vi "Format.vi"(8 "error in (no error)":errorcluster, 10 "LogRecord":refnum<class "LogRecord.lvclass">, 11 "DefaultLogFormat in":refnum<class "DefaultLogFormat.lvclass">) -> (0 "error out":errorcluster, 2 "Log Line":string, 3 "DefaultLogFormat out":refnum<class "DefaultLogFormat.lvclass">)   [LabVIEW 2024, in "DefaultLogFormat.lvclass"]
uses:
  DefaultLogFormat.lvclass
  Record/LogRecord.lvclass
  Record/LogRecord.lvclass/LogRecord.ctl
  DefaultLogFormat.lvclass/DefaultLogFormat.ctl
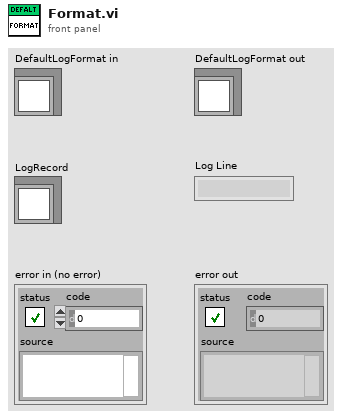
[diagram p1: front panel]
types:
  T1 = typedef "LoggerShared.lvlib/Level.ctl" = enum16{"DEBUG", "INFO", "WARNING", "ERROR", "CRITICAL"}
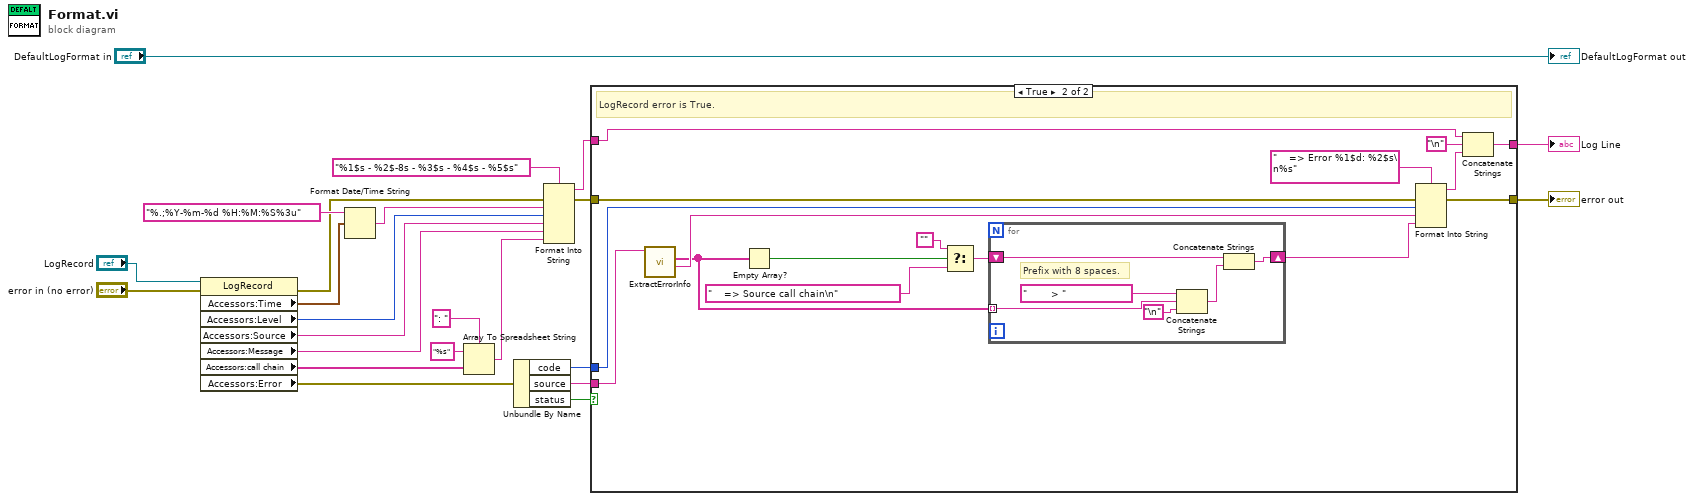
[diagram p0: block diagram]
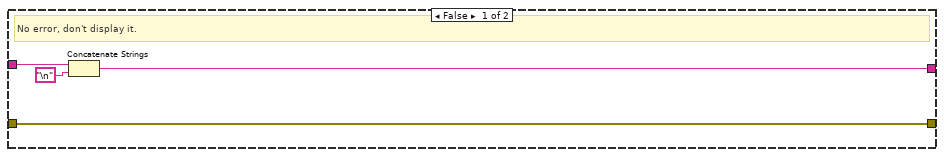
[diagram p2: hidden frame]
diagram:
  n1 = property class="LogRecord"(reference="LogRecord", error in="error in (no error)") -> (error out=w3:errorcluster, "Accessors:Time"=w20:timestamp, "Accessors:Level"=w17:T1, "Accessors:Source"=w16:string, "Accessors:Message"=w1:string, "Accessors:call chain"=w15:string[], "Accessors:Error"=w9:errorcluster)  [unwired: 1 out]
  n2 = Format Date/Time String(time format string (%c)="%.;%Y-%m-%d %H:%M:%S%3u" ("Datetime format"), seconds (now)=w20) -> (date/time string=w18:string)  [unwired: 1 in]
  n3 = Array To Spreadsheet String(delimiter (Tab)=": ", array=w15, 3:"%s" ("format string")) -> (spreadsheet string=w13:string)
  n4 = Unbundle By Name(w9) -> ("code"=w11:i32, "source"=w10:string, "status"=w12:bool)
  n5 = Format Into String(format string="%1$s - %2$-8s - %3$s - %4$s - %5$s" ("Log Line Format Specifier"), error in=w3, w18, w17, w16, w1, w13) -> (resulting string=w8:string, error out=w4:errorcluster)  [unwired: 1 in]
  n6 = case shown="True" w12 {
    tunnel: w11 -> [_ w43]
    tunnel: w10 -> [_ w37]
    tunnel: w8 -> [w27 w41]
    tunnel: w4 -> [w25 w42]
    tunnel: [w26 w39] -> w7
    tunnel: [w25 w38] -> w6
    frame False {
      # "No error, don't display it."
      n7 = Concatenate Strings(w27, "\n") -> (w26:string)
    }
    frame True {
      # "LogRecord error is True."
      n8 = call "ExtractErrorInfo.vi"("source in"=w37) -> ("result string"=w35:string, "Callchain"=w30:string[])  [unwired: 9 in]
      n9 = Empty Array?(array=w30) -> (empty?=w34:bool)
      n10 = Select(t="", s=w34, f="    => Source call chain\n") -> (s? t:f=w33:string)
      n11 = for {
        tunnel: w30 -> [w48] mode=indexing
        shift-right: [w45] -> w29
        shift-left: w33 -> [w47]
        # "Prefix with 8 spaces."
        n12 = Concatenate Strings("        > " ("string"), w48, "\n") -> (w46:string)
        n13 = Concatenate Strings(w47, w46) -> (w45:string)
      }
      n14 = Format Into String(format string="    => Error %1$d: %2$s\n%s" ("Error Line Format Specifier"), error in=w42, w43, w35, w29) -> (resulting string=w40:string, error out=w38:errorcluster)  [unwired: 1 in]
      n15 = Concatenate Strings(w41, "\n", w40) -> (w39:string)
    }
  }
  "error out" <- w6
  "Log Line" <- w7
  "DefaultLogFormat out" <- "DefaultLogFormat in"
